vi "Constants.vi"() -> ()   [LabVIEW 2020, in "AIM ARINC 664 Scripting.lvlib"]
doc: "Use this Global VI to access the GUIDs assigned to the page resources of the Custom Device."
uses:
  AIM ARINC 664 Scripting.lvlib
panel:
  in  "Tab Control":enum32{"GUIDs", "Constants", "Properties"}(tab)=enum."Constants"
  in  "GUID.Rx UDP Msg Count":string="20D2061A-1B55-4603-BB73-15A720A5F9F7"
  in  "GUID.Rx UDP Timestamp":string="F8FF7027-A744-45DE-B20E-B49377AF10BC"
  in  "GUID.Rx UDP Information":string="8CD308E2-B334-4A66-84D5-0ACA5E495365"
  in  "GUID.Rx Monitor Command Section":string="5D6E662D-4EFB-415B-AC3E-AA1F155779C7"
  in  "GUID.Tx Generic Command Section":string="2188B24A-3494-4477-93CF-25CD7C0BEFDF"
  in  "GUID.Sampling":string="B89465D2-793A-4104-A0ED-B169B72F9E43"
  in  "GUID.VL":string="AD8B37F3-F79C-4716-A9ED-786B96288466"
  in  "GUID.Tx UDP":string="85BBE12C-C4A9-4523-B3FC-3068DB103764"
  in  "GUID.Rx UDP":string="BD85F639-FFC8-443D-8B3E-A57AB37A5B2A"
  in  "GUID.Status Section":string="C7B8E643-DB53-4236-A1BD-67967F46ACD2"
  in  "GUID.Monitor Queue Size Distribution":string="9C3365A4-3BC6-46D2-9E4A-E79F510F5B35"
  in  "GUID.Monitor Queue Error":string="1B82B94F-FAA8-416B-810A-FCB6E86E6CD6"
  in  "GUID.Monitor Queue Utilization":string="D9396964-5902-4E2A-82C8-2A696FD85A36"
  in  "GUID.Logging Enable":string="F7E12D6B-92C4-4571-A0A0-26B66B4144B7"
  in  "GUID.Logging":string="F10A60DD-15A2-4C5A-ACFB-58AB9BD738ED"
  in  "GUID.Tx Generic":string="4DFFD447-F0AD-4072-98FE-86FA01F16D58"
  in  "GUID.Configuration File Page":string="C40B493B-66E6-407A-B069-3D0F2F03B0B0"
  in  "GUID.Main Page":string="E4CCF68F-8FD0-4415-8B77-04F5B0B8774E"
  in  "GUID.Monitor Queue Status Section":string="B887D8B9-C6CF-4F1C-8F75-15EFFDD5CFFC"
  in  "GUID.Queue Status Generic Channel":string="4F18D536-EE77-43DD-87DF-7965B9424EF3"
  in  "GUID.Tx Generic Status Section":string="C7869D6F-30D0-4274-87C5-5BE67BEEE020"
  in  "GUID.Timing":string="0B10B407-FC53-4972-B99A-2B34594513BC"
  in  "GUID.Disabled Custom Device":string="A66CC76D-6CC8-4007-ADC5-D1CC0A2F1CEE"
  in  "GUID.Channel":string="CF0CA23A-EB41-46AB-9644-A73D53E8CC9A"
  in  "GUID.Import Frames":string="91A9FDF9-5DFB-4541-8AF4-19D661EA6B3F"
  in  "GUID.Outgoing":string="84DDE259-6DAA-47F4-95FE-5FAF375E7F83"
  in  "GUID.Incoming":string="5B8531B6-763C-44A7-B58A-6C82ED2F2D56"
  in  "GUID.Database":string="65BC4E28-E356-47F9-BC1B-E791645CB113"
  in  "GUID.Add Database":string="B9E75FE6-03B9-4048-9BC0-825D89CA1CFB"
  in  "GUID.Port":string="582DDD9C-BC3D-4862-8B5A-626848E183CB"
  in  "GUID.Add Port":string="7014092B-3C0E-41CD-B0BA-E6BCDDEE50A9"
  in  "GUID.Databases":string="527460C4-E046-4BBC-87C1-693B28D30B6B"
  in  "GUID.Ports":string="A1D05803-877A-4AF1-8556-3AC960D2123E"
  in  "Protocol":string="DE983FBA-D8F6-4783-A85D-48BA014B4826"
  in  "Vendor":string="76E8A5AC-CC3C-4AA0-AEF7-C5961C7E330A"
  in  "GUID.Frame":string="E66E8388-7A61-4B6A-926A-BD76449CDED7"
  in  "GUID.Custom Device":string="E6D0F9EC-E47C-4FC9-91FD-2E458AB6A646"
  in  "Rx UDP Msg Error Count":string="Error Count"
  in  "Rx UDP Information":string="Information"
  in  "Rx UDP Msg Count":string="Count"
  in  "Rx UDP Timestamp":string="Timestamp"
  in  "Monitor Reset Mode":string="Reset Mode"
  in  "Monitor Reset Channel":string="RxStatus"
  in  "Tx Generic Enable Command":string="Enable Tx"
  in  "Tx Generic Command Section":string="Tx Generic Commands"
  in  "Tx UDP Status":string="Tx UDP Status"
  in  "Rx UDP Status":string="Rx UDP Status"
  in  "Tx UDP":string="Tx UDP"
  in  "Rx UDP":string="Rx UDP"
  in  "Status Section":string="Status"
  in  "Monitor Queue Status Size":string="Monitor Size Distribution"
  in  "Monitor Queue Status Error":string="Monitor Error"
  in  "Monitor Queue Status Utilization":string="Monitor Utilization"
  in  "Logging":string="Logging"
  in  "Tx Generic":string="Tx Generic"
  in  "Configuration File":string="Configuration File"
  in  "Rx MACLong Channel":string="MACLong"
  in  "Rx MAC1024To1518Count Channel":string="MAC1024To1518Count"
  in  "Rx MAC512To1023Count Channel":string="MAC512To1023Count"
  in  "Rx MAC256To511Count Channel":string="MAC256To511Count"
  in  "Rx MAC128To255Count Channel":string="MAC128To255Count"
  in  "Rx MAC64To127Count Channel":string="MAC64To127Count"
  in  "Rx MAC1Short Channel":string="MAC1Short"
  in  "Rx TrafShapingViolationCount Channel":string="TrafShapingViolationCount"
  in  "Rx SNIntegrityErrorCount Channel":string="SNIntegrityErrorCount"
  in  "Rx VLLenErrorCount Channel":string="VLLenErrorCount"
  in  "Rx NoSfdErrorCount Channel":string="NoSfdErrorCount"
  in  "Rx MACErrorCount Channel":string="MACErrorCount"
  in  "Rx IPErrorCount Channel":string="IPErrorCount"
  in  "Rx IFGErrorCount Channel":string="IFGErrorCount"
  in  "Rx CRCErrorCount Channel":string="CRCErrorCount"
  in  "Rx UnaligErrorCount Channel":string="UnaligErrorCount"
  in  "Rx PreamErrorCount Channel":string="PreamErrorCount"
  in  "Rx PhysErrorCount Channel":string="PhysErrorCount"
  in  "Rx FramesPerSecond Channel":string="FramesPerSecond"
  in  "Rx BytesPerSecond Channel":string="BytesPerSecond"
  in  "Rx FrameErrorCount Channel":string="FrameErrorCount"
  in  "Rx FrameGoodCount Channel":string="FrameGoodCount"
  in  "Rx TotalByteCount Channel":string="TotalByteCount"
  in  "Monitor RxStatus Channel":string="RxStatus"
  in  "Tx FramesPortB Channel":string="FramesPortB"
  in  "Tx TransmitMode Channel":string="TransmitMode"
  in  "Tx Frames Channel":string="Frames"
  in  "Tx Status Channel":string="Status"
  in  "Monitor BytesToRead Channel":string="BytesToRead"
  in  "Monitor FramesToRead Channel":string="FramesToRead"
  in  "Monitor QueueStatus Channel":string="QueueStatus"
  in  "Monitor Queue Status Section":string="Monitor"
  in  "Tx FramesInCycQueue Channel":string="FramesInCycQueue"
  in  "Tx FramesSent Channel":string="FramesSent"
  in  "Tx BytesReloadable Channel":string="BytesReloadable"
  in  "Tx QueueStatus Channel":string="QueueStatus"
  in  "Tx Generic Status Section":string="Tx Generic Status"
  in  "Timing":string="Timing"
  in  "Channel":string="Channel"
  in  "Frame":string="Frame"
  in  "Outgoing":string="Outgoing"
  in  "Incoming":string="Incoming"
  in  "Database":string="Database"
  in  "Port":string="Port"
  in  "Ports":string="Ports"
  in  "Logging.Enable":string="Enable Logging"
  in  "Rx Monitor Command Section":string="Rx Monitor Commands"
  in  "Outgoing Frame Rate":string="Outgoing Frame Rate"
  in  "Incoming Frame Rate":string="Incoming Frame Rate"
  in  "Inline Rx UDP":string="Inline Rx UDP"
  in  "Inline Tx UDP":string="Inline Tx UDP"
  in  "Inline Rx Monitor":string="Inline  Rx Monitor"
  in  "Inline Tx Generic":string="Inline Tx Generic"
  in  "RawFramePerPayload":string="Payload.RawFrameList"
  in  "PayloadMap":string="Payload.Map"
  in  "PayloadID":string="Payload.ID"
  in  "RawFrameMap":string="RawFrame.Map"
  in  "Prop.Segment Files By":string="Segment Files By"
  in  "Prop.Segmentation Threshold":string="Segmentation Threshold"
  in  "Prop.Disk Space Percentage":string="Disk Space Percentage"
  in  "Prop.Check Disk Space":string="Check Disk Space"
  in  "Prop.Segment File":string="Segment File"
  in  "PayloadFile.Path":string="PayloadFile.Path"
  in  "UDPFrameID":string="UDPFrame.ID"
  in  "Prop.Enable Logging":string="Enabled"
  in  "FrameArrayFile.Needed":string="FrameArrayFile.Needed"
  in  "ConfigurationFile.Needed":string="ConfigurationFile.Needed"
  in  "Tx.Generic.Path":string="Tx.Generic.Path"
  in  "XML.BoardID":string="BoardID"
  in  "ConfigurationFile.Path":string="ConfigurationFile.Path"
  in  "Database.Path":string="Database.Path"
  in  "Database.Name":string="Database.Name"
  in  "Frame.ID":string="Frame.ID"
  in  "Compiled.Settings":string="Compiled.Settings"
  in  "Prop.Logging.Directory":string="Log Directory"
  in  "Prop.Logging.BaseName":string="Base Name"
  in  "Prop.Logging.TimestampName":string="Timestamp"
  # "Not Used - Not deleted\nbecause it is in the framework"
  # "Board Properties"
  # "System"
  # "In Frame System but not used"
  # "Tx Generic Properties"
  # "Monitor Properties"
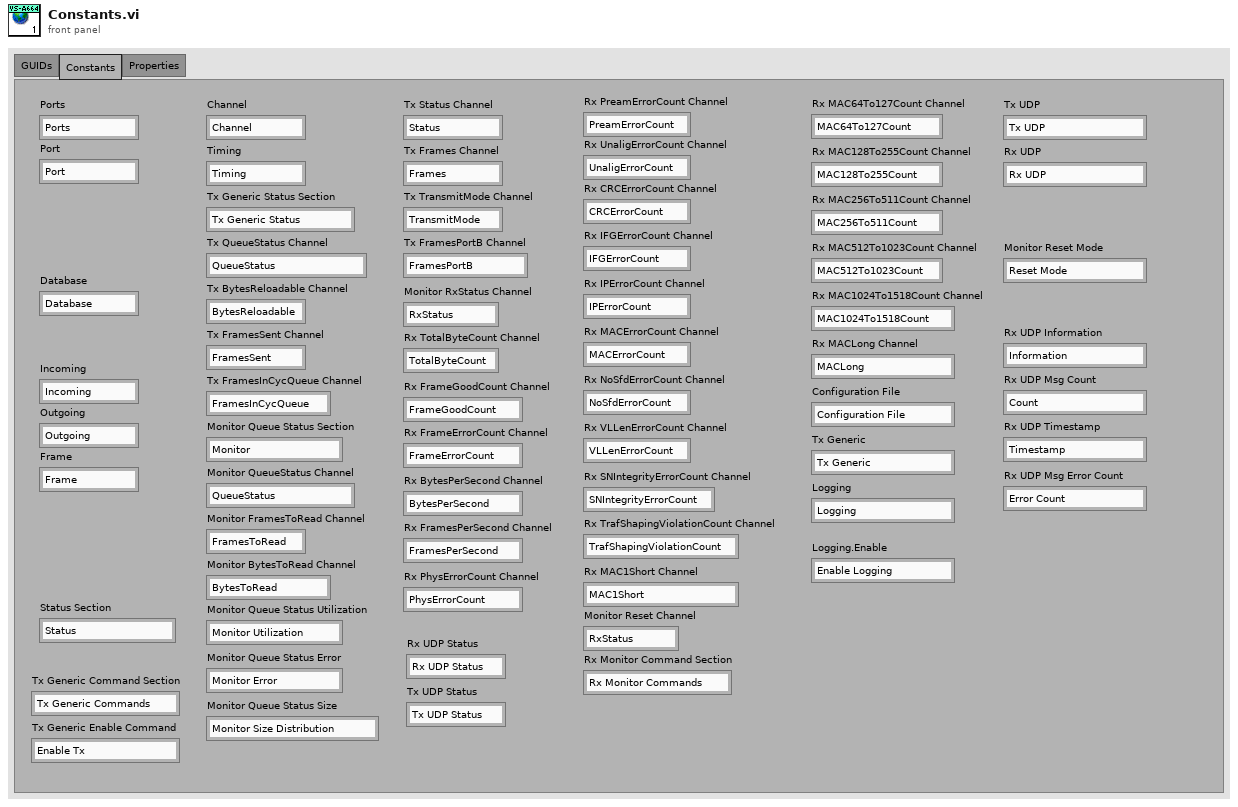
[diagram p1: front panel]
diagram:
